vi "RSZVB Set IMOD Enhanced Wave Correction.vi"(8 "error in (no error)":errorcluster {"code" format="%.0x"}, 9 "State (Off)":bool, 10 "Channel (1)":i32=1, 11 "VISA session":refnum<visa-resource-name>) -> (0 "error out":errorcluster {"code" format="%.0x"}, 3 "dup VISA session":refnum<visa-resource-name>)   [LabVIEW 2011]
doc: "This VI switches the preparation for an enhanced wave correction of an intermodulation measurement on or off. \n\nRemote-control command(s):\n[SENSe<Ch>:]FREQuency:IMODulation:PEWCorr[:STATe]"
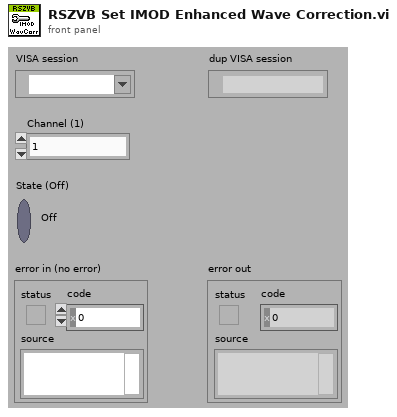
[diagram p1: front panel]
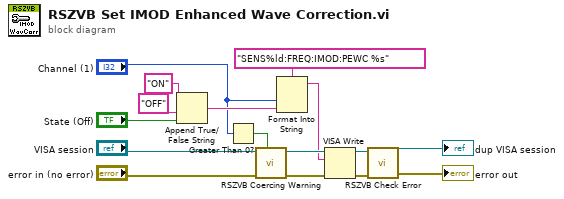
[diagram p0: block diagram]
diagram:
  n1 = Append True/False String(1:"State (Off)", 2:"OFF" ("false string"), 3:"ON" ("true string")) -> (0:w16:string)  [unwired: 1 in]
  n2 = Greater Than 0?(x="Channel (1)") -> (x > 0?=w8:bool)
  n3 = call "RSZVB Coercing Warning.vi"("In Range?"=w8, "error in (no error)"="error in (no error)", "VISA session"="VISA session") -> ("error out"=w9:errorcluster, "dup VISA session"=w10:refnum<visa-resource-name>)  [unwired: 7 in]
  n4 = Format Into String(format string="SENS%ld:FREQ:IMOD:PEWC %s", "Channel (1)", w16) -> (resulting string=w7:string)  [unwired: 2 in, 1 out]
  n5 = VISA Write(VISA resource name=w10, write buffer=w7, error in (no error)=w9) -> (VISA resource name out=w13:refnum<visa-resource-name>, error out=w12:errorcluster)  [unwired: 1 out]
  n6 = call "RSZVB Check Error.vi"("error in (no error)"=w12, "VISA session"=w13) -> ("error out"=→"error out":errorcluster, "dup VISA session"=→"dup VISA session":refnum<visa-resource-name>)  [unwired: 8 in]
